vi "Main.vi"() -> ()   [LabVIEW 2015]
uses:
  TypeAction1.ctl
  RS232_to_FPGA/RS232ToFPGA.lvlib
panel:
  out "element":T1
  in  "stop":bool
  in  "Tab Control":enum32{"FPGA Registers", "FPGA Coef"}(tab)
  in  "Registers":string[][](table)
  in  "Save":bool
  in  "Load":bool
  in  "TXT Configuration Path":path
  in  "Convert In Txt":bool
  out "Done":bool
  in  "Write Setting HW":bool
  in  "XML Configuration Path (RegisterMapEditor *.mmp)":path
  in  "Clear":bool
  in  "Number Reg":u16=26
  in  "Base Address":string
  in  "Load R/I":bool
  in  "Real File Path":path
  in  "Imaginary File Path":path
  out "Re/Img Coef":dbl[][](array[numeric])
  in  "Write Coeff":bool
  in  "Filtre":u16(ring) items=["Filter 0", "Filter 1", "Filter 2", "Filter 3"]
  out "Size Coef I/R":i32
  in  "error in":errorcluster
  out "error out":errorcluster
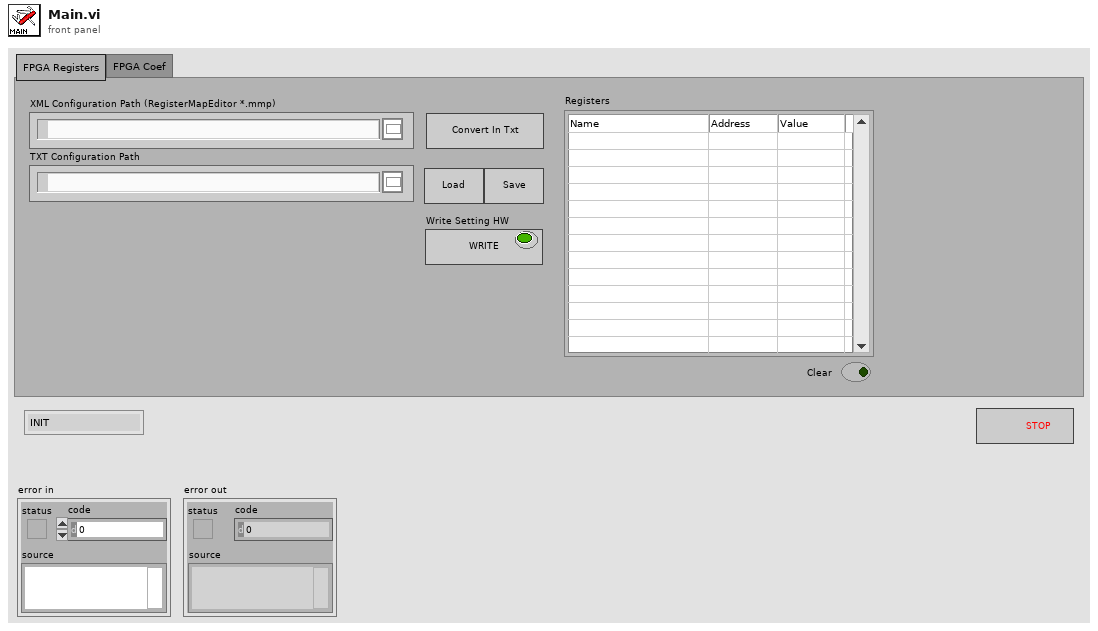
[diagram p1: front panel]
types:
  T1 = typedef "TypeAction1.ctl" = enum16{"INIT", "WriteSettingHW", "WriteSettingCoef", "ConvertToTxtFile", "SaveConfigTxt", "LoadConfigTxt", "LoadRICoef", "STOP"}
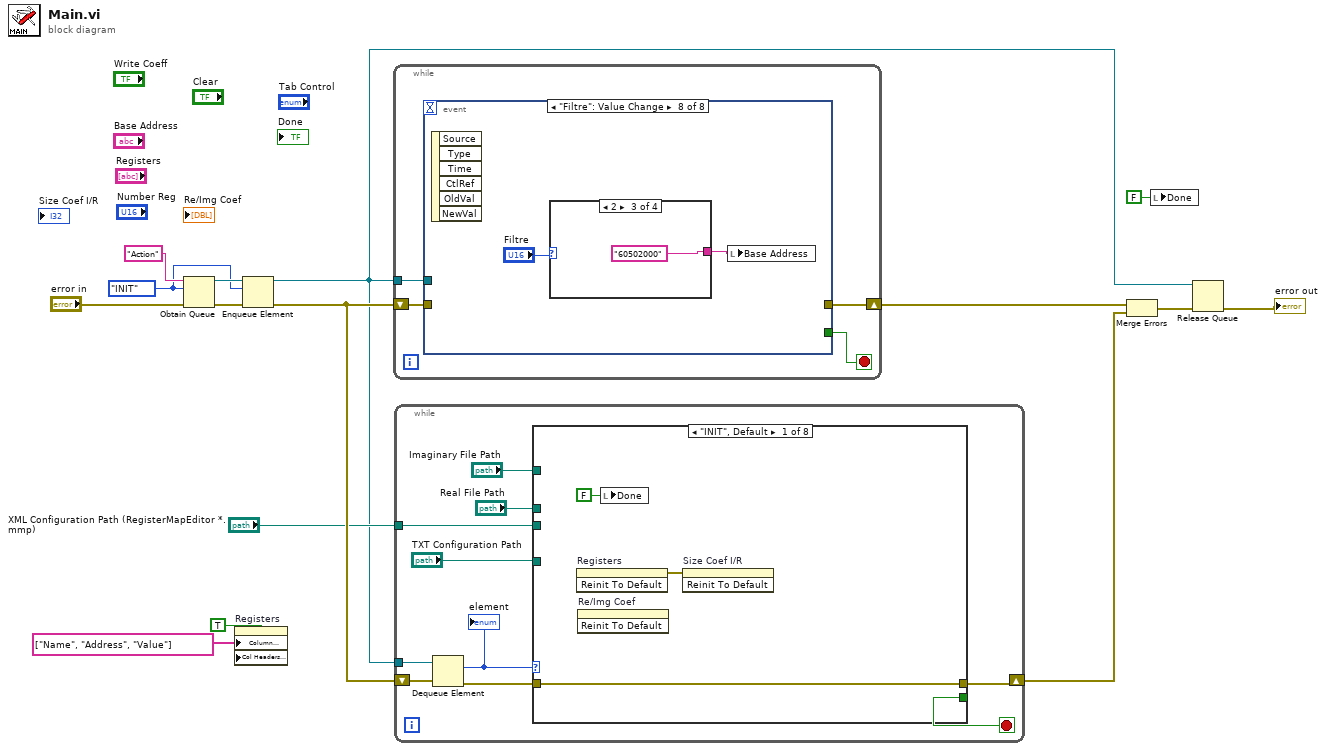
[diagram p0: block diagram]
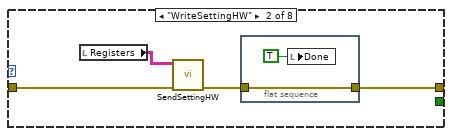
[diagram p2: hidden frame]
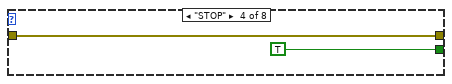
[diagram p4: hidden frame]
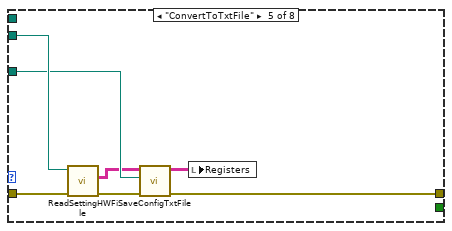
[diagram p5: hidden frame]
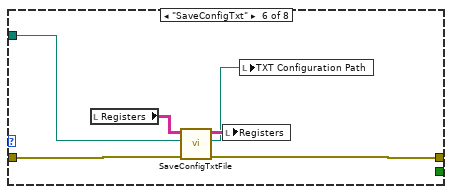
[diagram p6: hidden frame]
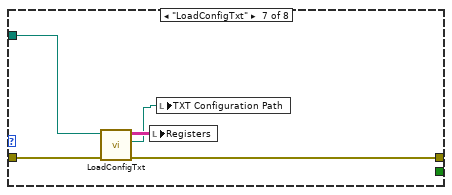
[diagram p7: hidden frame]
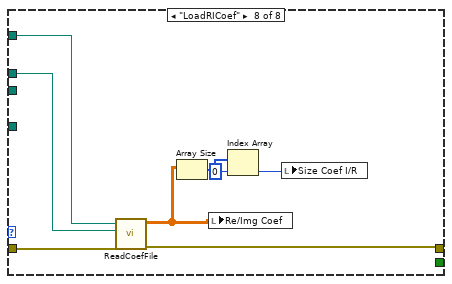
[diagram p8: hidden frame]
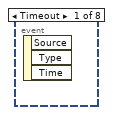
[diagram p9: hidden frame]
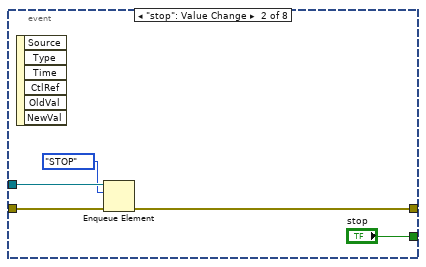
[diagram p10: hidden frame]
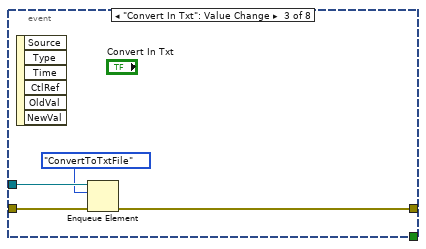
[diagram p11: hidden frame]
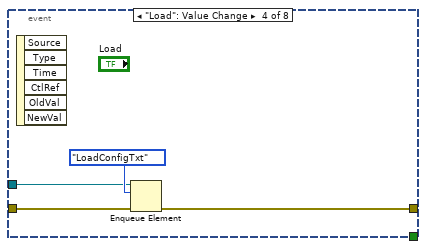
[diagram p12: hidden frame]
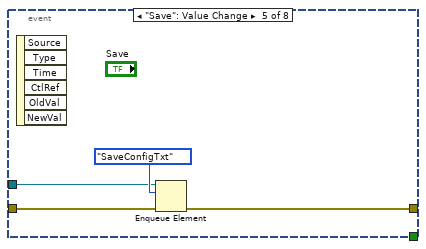
[diagram p13: hidden frame]
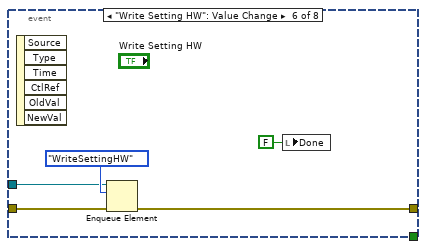
[diagram p14: hidden frame]
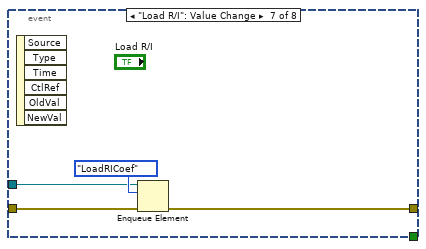
[diagram p15: hidden frame]
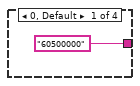
[diagram p16: hidden frame]
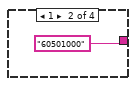
[diagram p17: hidden frame]
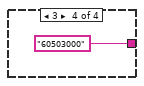
[diagram p18: hidden frame]
diagram:
  w11 = TypeAction1."INIT" ("Action")
  n1 = Obtain Queue(name (unnamed)="Action", element data type=w11, error in (no error)="error in") -> (queue out=w12:refnum<queue>, error out=w13:errorcluster)  [unwired: 2 in, 1 out]
  n2 = property on="Registers" class="Tbl (strict)"("Column Headers[]"=string[] ["Name", "Address", "Value"] ("Column Header Strings[]"), "Col Headers Vis"=TRUE ("Visible Items:Column Headers Visible")) -> ()  [unwired: 2 in, 2 out]
  n3 = Enqueue Element(queue=w12, element=w11, error in (no error)=w13) -> (queue out=w3:refnum<queue>, error out=w10:errorcluster)  [unwired: 1 in, 1 out]
  n4 = while {
    shift-right: [w17] -> w9
    shift-left: w10 -> [w19]
    tunnel: w3 -> [w18]
    stop <- w16 stop-if-true
    n5 = event shown="[7] \"Filtre\": Value Change" {
      selector: _ -> [_ _ _ _ _ _ _ _]
      dyn-events: _ -> [_ _ _ _ _ _ _ _]
      timeout: _ -> [_ _ _ _ _ _ _ _]
      tunnel: w19 -> [_ w24 w28 w31 w34 w40 w45 _]
      tunnel: w18 -> [_ w23 w26 w30 w35 w38 w42 _]
      tunnel: [_ w21 w27 w29 w33 w39 w44 _] -> w17
      tunnel: [_ "stop" _ _ _ _ _ _] -> w16
      event Timeout {
        n6 = event-data() -> ()  [unwired: 1 in, 3 out]
      }
      event "stop": Value Change {
        n7 = event-data() -> ()  [unwired: 1 in, 6 out]
        n8 = Enqueue Element(queue=w23, element=TypeAction1."STOP" ("Action"), error in (no error)=w24) -> (error out=w21:errorcluster)  [unwired: 1 in, 2 out]
      }
      event "Convert In Txt": Value Change {
        n9 = event-data() -> ()  [unwired: 1 in, 6 out]
        n10 = Enqueue Element(queue=w26, element=TypeAction1."ConvertToTxtFile", error in (no error)=w28) -> (error out=w27:errorcluster)  [unwired: 1 in, 2 out]
      }
      event "Load": Value Change {
        n11 = event-data() -> ()  [unwired: 1 in, 6 out]
        n12 = Enqueue Element(queue=w30, element=TypeAction1."LoadConfigTxt" ("Action"), error in (no error)=w31) -> (error out=w29:errorcluster)  [unwired: 1 in, 2 out]
      }
      event "Save": Value Change {
        n13 = event-data() -> ()  [unwired: 1 in, 6 out]
        n14 = Enqueue Element(queue=w35, element=TypeAction1."SaveConfigTxt" ("Action"), error in (no error)=w34) -> (error out=w33:errorcluster)  [unwired: 1 in, 2 out]
      }
      event "Write Setting HW": Value Change {
        n15 = event-data() -> ()  [unwired: 1 in, 6 out]
        n16 = Enqueue Element(queue=w38, element=TypeAction1."WriteSettingHW" ("Action"), error in (no error)=w40) -> (error out=w39:errorcluster)  [unwired: 1 in, 2 out]
        n17 = local write "Done"(FALSE ("Done")) -> ()
      }
      event "Load R/I": Value Change {
        n18 = event-data() -> ()  [unwired: 1 in, 6 out]
        n19 = Enqueue Element(queue=w42, element=TypeAction1."LoadRICoef" ("Action"), error in (no error)=w45) -> (error out=w44:errorcluster)  [unwired: 1 in, 2 out]
      }
      event "Filtre": Value Change {
        n20 = event-data() -> ()  [unwired: 1 in, 6 out]
        n21 = case shown="2" "Filtre" {
          tunnel: ["60500000" "60501000" "60502000" "60503000"] -> w46
          frame 0, Default {
          }
          frame 1 {
          }
          frame 2 {
          }
          frame 3 {
          }
        }
        n22 = local write "Base Address"(w46) -> ()
      }
    }
  }
  n23 = while {
    tunnel: w3 -> [w61]
    tunnel: "XML Configuration Path (RegisterMapEditor *.mmp)" -> [w56]
    shift-right: [w57] -> w8
    shift-left: w10 -> [w60]
    stop <- w58 stop-if-true
    n24 = Dequeue Element(queue=w61, error in (no error)=w60) -> (element=w59:T1, error out=w55:errorcluster)  [unwired: 1 in, 2 out]
    "element" <- w59
    n25 = case shown="\"INIT\", Default" w59 {
      tunnel: [_ _ _ TRUE _ _ _ _] -> w58
      tunnel: [w64 w66 _ w71 w76 w84 w89 w97] -> w57
      tunnel: w55 -> [w64 w68 _ w71 w79 w85 w90 w98]
      tunnel: w56 -> [_ _ _ _ w78 _ _ _]
      tunnel: "TXT Configuration Path" -> [_ _ _ _ w75 w83 w87 _]
      tunnel: "Real File Path" -> [_ _ _ _ _ _ _ w96]
      tunnel: "Imaginary File Path" -> [_ _ _ _ _ _ _ w95]
      frame "INIT", Default {
        n26 = invoke on="Registers" class="Tbl (strict)" method="Reinit To Default"() -> (error out=w62:errorcluster)  [unwired: 3 in, 2 out]
        n27 = invoke on="Re/Img Coef" class="Arr (strict)" method="Reinit To Default"() -> ()  [unwired: 3 in, 3 out]
        n28 = local write "Done"(FALSE ("Done")) -> ()
        n29 = invoke on="Size Coef I/R" class="DigNum (strict)" method="Reinit To Default"(error in=w62) -> ()  [unwired: 2 in, 3 out]
      }
      frame "WriteSettingHW" {
        n30 = local read "Registers"() -> (w65:string[][])
        n31 = call "SendSettingHW.vi"("error in"=w68, "Data in"=w65) -> ("error out"=w67:errorcluster)  [unwired: 9 in]
        n32 = flat-sequence {
          tunnel: w67 -> [w69]
          tunnel: [w69] -> w66
          frame #0 {
            n33 = local write "Done"(TRUE ("Done")) -> ()
          }
        }
      }
      frame "WriteSettingCoef" {
      }
      frame "STOP" {
      }
      frame "ConvertToTxtFile" {
        n34 = call "ReadSettingHWFile.vi"("error in (no error)"=w79, "XML File Path"=w78) -> ("error out"=w77:errorcluster, "SettingRegister"=w74:string[][])  [unwired: 7 in, 1 out]
        n35 = call "SaveConfigTxtFile.vi"("error in"=w77, "file path (dialog if empty)"=w75, "Data in"=w74) -> ("error out"=w76:errorcluster, "Data out"=w73:string[][])  [unwired: 6 in, 1 out]
        n36 = local write "Registers"(w73) -> ()
      }
      frame "SaveConfigTxt" {
        n37 = local read "Registers"() -> (w81:string[][])
        n38 = call "SaveConfigTxtFile.vi"("error in"=w85, "file path (dialog if empty)"=w83, "Data in"=w81) -> ("error out"=w84:errorcluster, "file path"=w80:path, "Data out"=w82:string[][])  [unwired: 6 in]
        n39 = local write "Registers"(w82) -> ()
        n40 = local write "TXT Configuration Path"(w80) -> ()
      }
      frame "LoadConfigTxt" {
        n41 = call "LoadConfigTxt.vi"("error in"=w90, "file path (dialog if empty)"=w87) -> ("error out"=w89:errorcluster, "Path"=w86:path, "Data out"=w88:string[][])  [unwired: 7 in]
        n42 = local write "Registers"(w88) -> ()
        n43 = local write "TXT Configuration Path"(w86) -> ()
      }
      frame "LoadRICoef" {
        n44 = call "ReadCoefFile.vi"("error in"=w98, "Path Real in"=w96, "Path imaginary in"=w95) -> ("error out"=w97:errorcluster, "Real"=w92:dbl[][])  [unwired: 7 in]
        n45 = Array Size(array=w92) -> (size(s)=w94:i32[])
        n46 = local write "Re/Img Coef"(w92) -> ()
        n47 = Index Array(array=w94, index=0) -> (element=w91:i32)
        n48 = local write "Size Coef I/R"(w91) -> ()
      }
    }
  }
  n49 = Merge Errors(w9, w8) -> (w7:errorcluster)
  n50 = local write "Done"(FALSE ("Done")) -> ()
  n51 = Release Queue(queue=w3, error in (no error)=w7) -> (error out=→"error out":errorcluster)  [unwired: 1 in, 2 out]
